vi "R2 Time SBR Cycle.vi"(10 "Pump Status Array":bool[][](array[boolean])=[[TRUE, FALSE, TRUE, FALSE, FALSE], [TRUE, FALSE, FALSE, FALSE, TRUE], [FALSE, FALSE, FALSE, TRUE, FALSE], [FALSE, FALSE, FALSE, FALSE, FALSE], [FALSE, TRUE, FALSE, FALSE, FALSE], [FALSE, FALSE, FALSE, FALSE, FALSE]], 11 "Timing Array":u32[](array[numeric])=[80, 0, 25, 60, 5]) -> ()   [LabVIEW 2016]
uses:
  R2 Pump Manual Control.ctl
  R2Variables.lvlib
panel:
  in  "stop":bool
  out "Phase":dbl
  # "Call from Control.vi"
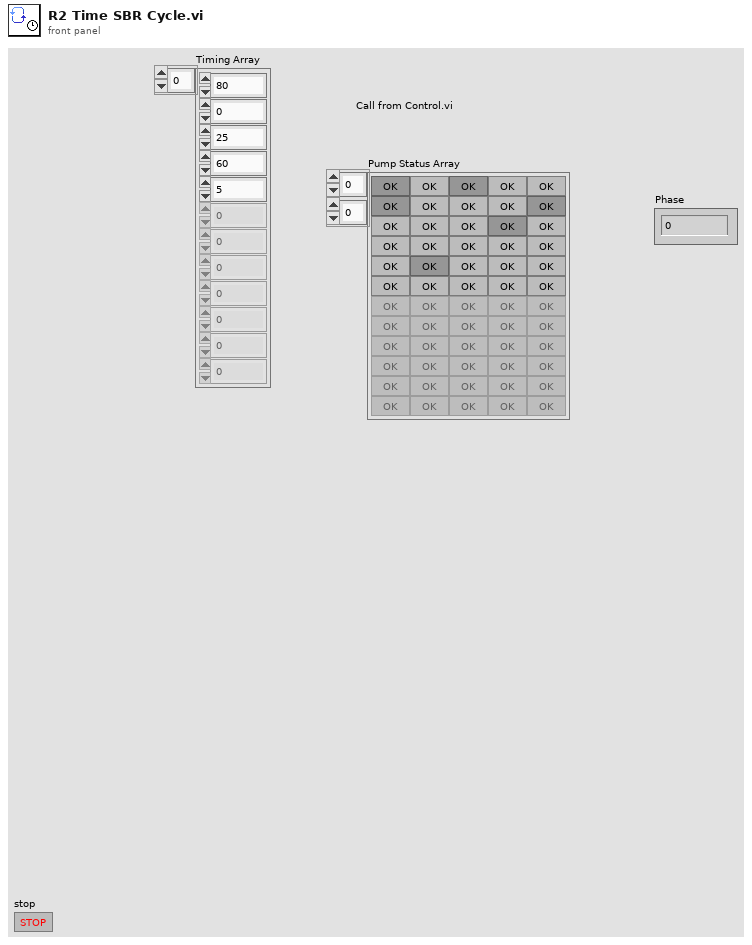
[diagram p1: front panel]
types:
  T1 = typedef "R2Variables.lvlib/R2 Pump Manual Control.ctl" = cluster{"Water Pump":bool, "Effluent Pump":bool, "Media Pump":bool, "Gas Pump":bool, "Air Release Valve":bool}
  T2 = cluster{"Pump Status Array[0]":bool, "Pump Status Array[1]":bool, "Pump Status Array[2]":bool, "Pump Status Array[3]":bool, "Pump Status Array[4]":bool, "Pump Status Array[5]":bool, "Pump Status Array[6]":bool, "Pump Status Array[7]":bool, "Pump Status Array[8]":bool}
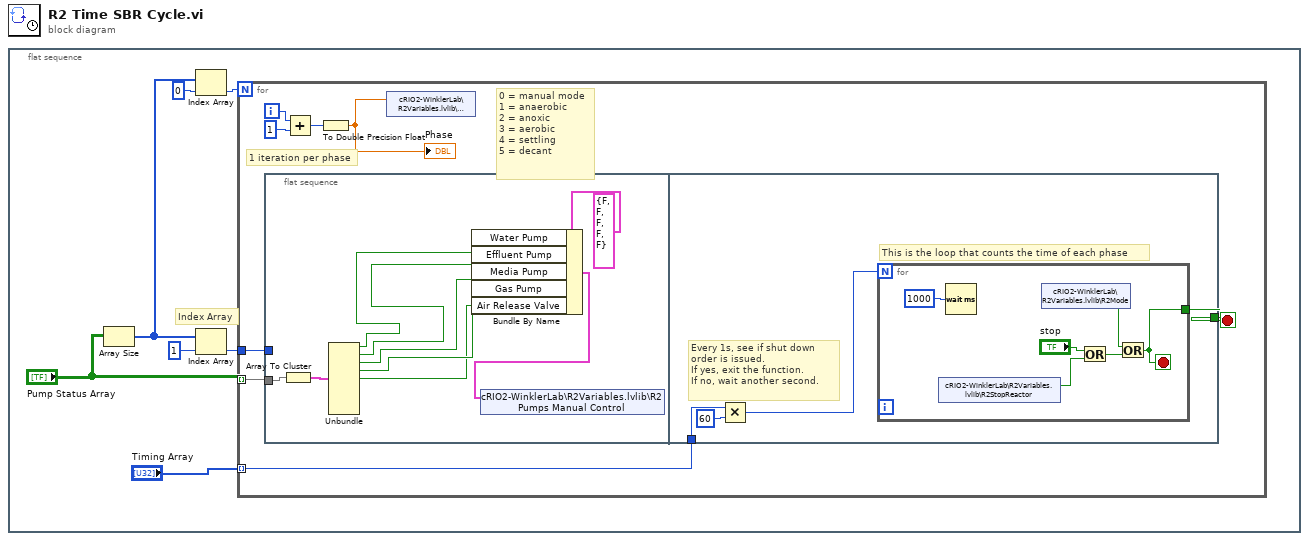
[diagram p0: block diagram]
diagram:
  n1 = flat-sequence {
    frame #0 {
      # "Index Array"
      n2 = Array Size(array="Pump Status Array") -> (size(s)=w5:i32[])
      n3 = Index Array(array=w5, index=0) -> (element=w2:i32)
      n4 = Index Array(array=w5, index=1) -> (element=w6:i32)
      n5 = for {
        N: w2 -> [_]
        tunnel: "Timing Array" -> [w13] mode=indexing
        tunnel: w6 -> [w15]
        tunnel: "Pump Status Array" -> [w14] mode=indexing
        i -> [w12]
        stop <- w8 stop-if-true
        # "0 = manual mode\n1 = anaerobic\n2 = anoxic\n3 = aerobic\n4 = settling\n5 = decant"
        # "1 iteration per phase"
        n6 = flat-sequence {
          tunnel: w15 -> [_]
          tunnel: w14 -> [w24]
          tunnel: w13 -> [w27]
          tunnel: [w26] -> w8
          frame #0 {
            n7 = Array To Cluster(array=w24) -> (cluster=w23:T2)
            n8 = Unbundle(w23) -> ("Pump Status Array[0]"=w21:bool, "Pump Status Array[1]"=w20:bool, "Pump Status Array[2]"=w19:bool, "Pump Status Array[3]"=w18:bool, "Pump Status Array[4]"=w17:bool)  [unwired: 4 out]
            n9 = Bundle By Name(cluster=T1 {"Water Pump"=FALSE, "Effluent Pump"=FALSE, "Media Pump"=FALSE, "Gas Pump"=FALSE, "Air Release Valve"=FALSE} ("Reactor 2 SBR Control"), "Water Pump"=w21, "Effluent Pump"=w20, "Media Pump"=w19, "Gas Pump"=w18, "Air Release Valve"=w17) -> (w16:T1)
            n10 = shared-variable "cRIO2-WinklerLab\\R2Variables.lvlib\\R2 Pumps Manual Control"(w16) -> ()  [unwired: 1 in, 1 out]
          }
          frame #1 {
            # "This is the loop that counts the time of each phase"
            # "Every 1s, see if shut down order is issued.\nIf yes, exit the function.\nIf no, wait another second."
            n11 = Multiply(x=w27, y=u32 60) -> (x*y=w25:u32)
            n12 = for {
              N: w25 -> [_]
              tunnel: [w30] -> w26
              stop <- w30 stop-if-true
              n13 = shared-variable "cRIO2-WinklerLab\\R2Variables.lvlib\\R2StopReactor"() -> (w29:bool)  [unwired: 1 in, 1 out]
              n14 = Wait (ms)(milliseconds to wait=u32 1000) -> ()  [unwired: 1 out]
              n15 = shared-variable "cRIO2-WinklerLab\\R2Variables.lvlib\\R2Mode"() -> (w31:bool)  [unwired: 1 in, 1 out]
              n16 = Or(x="stop", y=w29) -> (x .or. y?=w32:bool)
              n17 = Or(x=w31, y=w32) -> (x .or. y?=w30:bool)
            }
          }
        }
        n18 = Add(x=w12, y=1) -> (x+y=w10:i32)
        n19 = To Double Precision Float(number=w10) -> (double precision float=w9:dbl)
        "Phase" <- w9
        n20 = shared-variable "cRIO2-WinklerLab\\R2Variables.lvlib\\R2Phase"(w9) -> ()  [unwired: 1 in, 1 out]
      }
    }
  }
